vi "定制时间标识符.vi"() -> ()   [LabVIEW 2012]
panel:
  out "自定义时间格式":string
  out "时间标识字符串":string
  out "格式字符串":string
  out "时间标识":timestamp
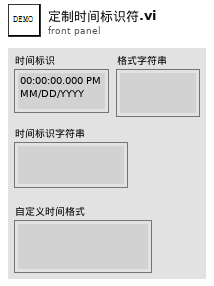
[diagram p1: front panel]
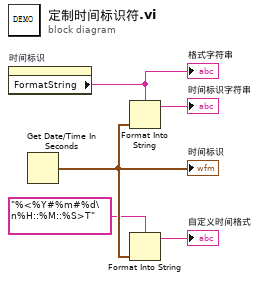
[diagram p0: block diagram]
diagram:
  n1 = property on="时间标识" class="AbsTime (严格)"() -> ("FormatString"=w5:string)  [unwired: 2 in, 2 out]
  "格式字符串" <- w5
  n2 = Get Date/Time In Seconds() -> (seconds since 1Jan1904=w3:timestamp)
  "时间标识" <- w3
  n3 = Format Into String(format string=w5, w3) -> (resulting string=→"时间标识字符串":string)  [unwired: 2 in, 1 out]
  n4 = Format Into String(format string="%<%Y#%m#%d\n%H::%M::%S>T" ("格式字符串"), w3) -> (resulting string=→"自定义时间格式":string)  [unwired: 2 in, 1 out]
